vi "TestWrite.vi"() -> ()   [LabVIEW 2019]
panel:
  out "Array 2":dbl[][](array[numeric])
  in  "Stop":bool
  in  "file path":path
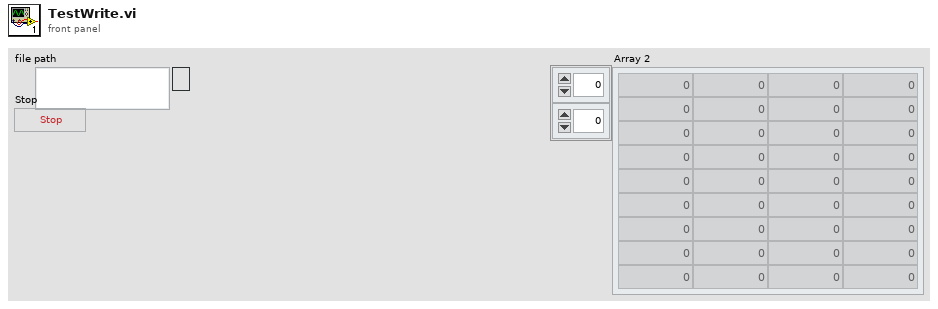
[diagram p1: front panel]
types:
  T1 = enum16{"open", "open or create", "create or replace", "create", "open (read-only)"}
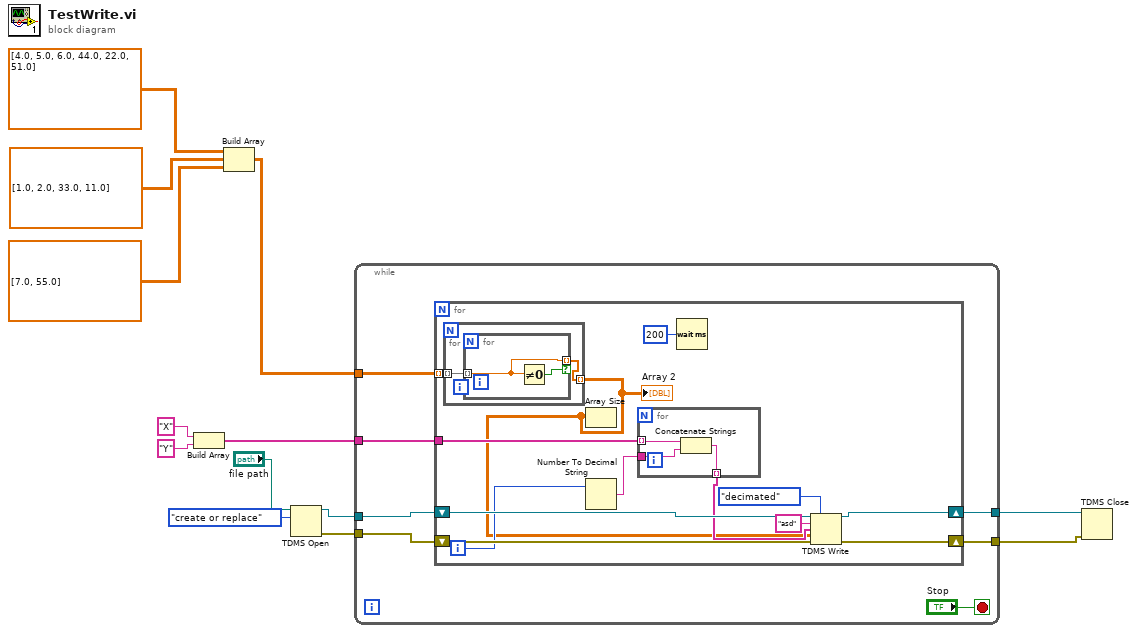
[diagram p0: block diagram]
diagram:
  n1 = Build Array("X", "Y") -> (w1:string[])
  n2 = Build Array(dbl[][] [[4.0, 5.0, 6.0], [44.0, 22.0, 51.0]], dbl[][] [[1.0, 2.0], [33.0, 11.0]], dbl[][] [[7.0], [55.0]]) -> (w4:dbl[][][])
  n3 = TDMS Open(10:T1."create or replace" ("operation (0:open)"), 11:"file path") -> (0:w10:errorcluster, 3:w11:refnum<k34>)  [unwired: 5 in]
  n4 = while {
    tunnel: w11 -> [w20]
    tunnel: w10 -> [w19]
    tunnel: [w18] -> w9
    tunnel: [w17] -> w8
    tunnel: w4 -> [w15]
    tunnel: w1 -> [w14]
    stop <- "Stop" stop-if-true
    n5 = for {
      shift-right: [w30] -> w17
      shift-left: w20 -> [w33]
      shift-right: [w31] -> w18
      shift-left: w19 -> [w32]
      tunnel: w15 -> [w22] mode=indexing
      tunnel: w14 -> [w26]
      i -> [w27]
      n6 = for {
        tunnel: w22 -> [w35] mode=indexing
        tunnel: [w34] -> w21 mode=indexing
        n7 = for {
          tunnel: w35 -> [w37] mode=indexing
          tunnel: [w37] -> w34 mode=indexing if=w36
          n8 = Not Equal To 0?(x=w37) -> (x != 0?=w36:bool)
        }
      }
      "Array 2" <- w21
      n9 = Array Size(array=w21) -> ()  [unwired: 1 out]
      n10 = Number To Decimal String(number=w27) -> (decimal integer string=w25:string)  [unwired: 1 in]
      n11 = for {
        tunnel: w26 -> [w40] mode=indexing
        tunnel: w25 -> [w39]
        tunnel: [w38] -> w24 mode=indexing
        n12 = Concatenate Strings(w40, w39) -> (w38:string)
      }
      n13 = Wait (ms)(milliseconds to wait=u32 200) -> ()  [unwired: 1 out]
      n14 = TDMS Write(0:w33, 1:enum16{"decimated", "interleaved"}."decimated" ("data layout (0:decimated)"), 5:"asd" ("group name in (Untitled)"), 7:w24, 9:w21, 11:w32) -> (4:w30:refnum<k34>, 15:w31:errorcluster)  [unwired: 2 out]
    }
  }
  n15 = TDMS Close(8:w9, 11:w8) -> ()  [unwired: 2 out]
